vi "Version_2.0_Single_Column_Code.vi"() -> ()   [LabVIEW 2020] (continued)
                                n5689 = Subtract(x=w6119, y=w6118) -> (x-y=w6117:dbl)
                                n5690 = Absolute Value(x=w6117) -> (abs(x)=w6116:dbl)
                                n5691 = Multiply(x=w6116, y=w6115) -> (x*y=w6114:dbl)
                                n5692 = Divide(x=w6114, y=3000.0) -> (x/y=w6112:dbl)
                                }
                                frame "High Resolution Pumping".. {
                                n5693 = Subtract(x=w6127, y=w6126) -> (x-y=w6125:dbl)
                                n5694 = Absolute Value(x=w6125) -> (abs(x)=w6124:dbl)
                                n5695 = Multiply(x=w6124, y=w6123) -> (x*y=w6122:dbl)
                                n5696 = Divide(x=w6122, y=24000.0) -> (x/y=w6120:dbl)
                                }
                                }
                                n5697 = local write "True Volume being \ninjected in this\nprocess"(w6106) -> ()
                                }
                                frame #1 {
                                # "From here on 'Volume being injected \nin this process' represents the volume \nin this sub process"
                                n5698 = call "AbsolutePlungerPosition (SubVI).vi"("VISA Refnum in"=w6133) -> ("Plunger Position"=w6131:i32)  [unwired: 10 in]
                                n5699 = case shown="..\"Standard Pumping\"" w6132 {
                                tunnel: w6131 -> [w6141 w6149]
                                tunnel: w6128 -> [w6140 w6148]
                                tunnel: w6130 -> [w6137 w6145]
                                tunnel: [w6134 w6142] -> w6129
                                frame .."Standard Pumping" {
                                n5700 = Subtract(x=w6141, y=w6140) -> (x-y=w6139:dbl)
                                n5701 = Absolute Value(x=w6139) -> (abs(x)=w6138:dbl)
                                n5702 = Multiply(x=w6138, y=w6137) -> (x*y=w6136:dbl)
                                n5703 = Divide(x=w6136, y=3000.0) -> (x/y=w6134:dbl)
                                }
                                frame "High Resolution Pumping".. {
                                n5704 = Subtract(x=w6149, y=w6148) -> (x-y=w6147:dbl)
                                n5705 = Absolute Value(x=w6147) -> (abs(x)=w6146:dbl)
                                n5706 = Multiply(x=w6146, y=w6145) -> (x*y=w6144:dbl)
                                n5707 = Divide(x=w6144, y=24000.0) -> (x/y=w6142:dbl)
                                }
                                }
                                n5708 = local write "Volume being Injected \nin this process"(w6129) -> ()
                                }
                                frame #2 {
                                n5709 = local read "Discard Volume"() -> (w6153:dbl)
                                n5710 = local read "Discard fluid \nprior to 1st \ndeposition"() -> (w6158:bool)
                                n5711 = local read "Volume being Injected \nin this process"() -> (w6157:dbl)
                                n5712 = Greater Or Equal?(x=w6157, y=w6153) -> (x >= y?=w6155:bool)
                                n5713 = call "AbsolutePlungerPositionStatus (SubVI).vi"("VISA Refnum in"=w6165) -> ("read buffer"=w6164:string)  [unwired: 10 in]
                                n5714 = local read "Stop for End of \nExperiment \nand Data Writing"() -> (w6152:bool)
                                n5715 = call <vilib>:"Trim Whitespace.vi"("string"=w6164) -> ("trimmed string"=w6163:string)  [unwired: 1 in]
                                n5716 = Not(x=w6158) -> (.not. x?=w6156:bool)
                                n5717 = Equal?(x=w6163, y="/0`\u0003") -> (x = y?=w6161:bool)
                                n5718 = Or(x=w6156, y=w6155) -> (x .or. y?=w6154:bool)
                                n5719 = local read "Re-SEC"() -> (w6151:bool)
                                n5720 = Or(x=w6152, y=w6151) -> (x .or. y?=w6150:bool)
                                n5721 = Or(x=w6154, y=w6150) -> (x .or. y?=w6160:bool)
                                n5722 = Or(x=w6161, y=w6160) -> (x .or. y?=w6159:bool)
                                }
                                }
                                n5723 = Wait (ms)(milliseconds to wait=u32 100) -> ()  [unwired: 1 out]
                                }
                                n5724 = local write "Valve V4 Open"(TRUE ("Valve V4 Open")) -> ()
                                n5725 = local write "Valve V3 Open"(TRUE ("Valve V3 Open")) -> ()
                                n5726 = local write "Valve V2 Open"(FALSE ("Valve V2 Open")) -> ()
                                n5727 = local write "Valve V1 Open"(FALSE ("Valve V1 Open")) -> ()
                                n5728 = local write "External Valve \nOpen"(FALSE ("External Valve \nOpen")) -> ()
                                n5729 = local write "Valve V5 Open"(TRUE ("Valve V5 Open")) -> ()
                                n5730 = local write "Valve V6 Open"(TRUE ("Valve V6 Open")) -> ()
                                n5731 = local write "Valve V8 Open"(FALSE ("Valve V8 Open")) -> ()
                                n5732 = local write "Valve V7 Open"(FALSE ("Valve V7 Open")) -> ()
                                n5733 = local write "Volume being Injected \nin this process"(0.0) -> ()
                                }
                                frame #1 {
                                # "Keeps the on-chip valve V1, V2 and V3 closed,\nHalts also deposition onto the grid\nand waits for the 1st redeposit command. Once the command is issued\nit starts pumpoing and moves onto the next frame"
                                n5734 = stacked-sequence {
                                frame #0 {
                                n5735 = local write "Valve V5 Open"(FALSE ("Valve V5 Open")) -> ()
                                n5736 = local write "Valve V1 Open"(FALSE ("Valve V1 Open")) -> ()
                                n5737 = local read "VISA Refnum in\nfor Pump"() -> (w6177:refnum<visa-resource-name>)
                                n5738 = local write "Valve V2 Open"(FALSE ("Valve V2 Open")) -> ()
                                n5739 = local write "Valve V6 Open"(FALSE ("Valve V6 Open")) -> ()
                                n5740 = local write "Re-deposit Sample\nonto Grid"(FALSE ("Redeposit Sample\nonto Grid")) -> ()
                                n5741 = local write "Pause Data Collection"(TRUE ("Pause Data Collection")) -> ()
                                n5742 = call "HardStopCurrentProcess (SubVI).vi"("VISA Refnum in"=w6177) -> ()  [unwired: 11 in]
                                n5743 = local write "Valve V7 Open"(FALSE ("Valve V7 Open")) -> ()
                                n5744 = local write "Valve V3 Open"(FALSE ("Valve V3 Open")) -> ()
                                n5745 = local write "External Valve \nOpen"(FALSE ("External Valve \nOpen")) -> ()
                                n5746 = local write "Valve V4 Open"(FALSE ("Valve V4 Open")) -> ()
                                n5747 = local write "Valve V8 Open"(FALSE ("Valve V8 Open")) -> ()
                                }
                                frame #1 {
                                n5748 = while {
                                stop <- w6183 stop-if-true
                                n5749 = local read "Stop for End of \nExperiment \nand Data Writing"() -> (w6181:bool)
                                n5750 = local read "Re-SEC"() -> (w6182:bool)
                                n5751 = local read "Re-deposit Sample\nonto Grid"() -> (w6184:bool)
                                n5752 = Or(x=w6181, y=w6182) -> (x .or. y?=w6180:bool)
                                n5753 = Or(x=w6184, y=w6180) -> (x .or. y?=w6183:bool)
                                }
                                n5754 = local write "Discard fluid \nprior to 1st \ndeposition"(FALSE ("Discard fluid \nprior to 1st \ndeposition")) -> ()
                                n5755 = One Button Dialog(message="Do you want to deposit sample on another grid? If yes, turn on 'Re-deposit Sample onto Grid'. Else turn on Re-SEC to do SEC again or STOP to end the experiment") -> ()  [unwired: 1 in, 1 out]
                                }
                                frame #2 {
                                n5756 = local write "Valve V6 Open"(TRUE ("Valve V3 Open")) -> ()
                                n5757 = local write "Valve V4 Open"(TRUE ("Valve V1 Open")) -> ()
                                n5758 = local write "Valve V5 Open"(TRUE ("Valve V2 Open")) -> ()
                                n5759 = local write "Valve V3 Open"(TRUE ("Valve V3 Open")) -> ()
                                n5760 = local write "Valve V7 Open"(FALSE ("Valve V7 Open")) -> ()
                                }
                                frame #3 {
                                n5761 = local read "Re-deposit Sample\nonto Grid"() -> (w6190:bool)
                                n5762 = case shown="True" w6190 {
                                frame False {
                                n5763 = local write "Suction On/Off"(FALSE ("Suction On/Off")) -> ()
                                }
                                frame True {
                                n5764 = stacked-sequence {
                                frame #0 {
                                n5765 = local read "VISA Refnum in\nfor Pump"() -> (w6193:refnum<visa-resource-name>)
                                n5766 = call "AbsolutePlungerPosition (SubVI).vi"("VISA Refnum in"=w6193) -> ("Plunger Position"=w6192:i32)  [unwired: 10 in]
                                n5767 = local write "Position\nNow"(w6192) -> ()
                                }
                                frame #1 {
                                n5768 = local read "Buffer-C2 Pumping\nResolution"() -> (w6195:T2)
                                n5769 = case shown="\"Standard Pumping\", Default" w6195 {
                                tunnel: [w6196 w6207] -> w6194
                                frame "Standard Pumping", Default {
                                n5770 = local read "Buffer-C2 Volume \nto be Pumped"() -> (w6199:dbl)
                                n5771 = local read "Volume of Syringe"() -> (w6202:dbl)
                                n5772 = local read "Initial Plunger Position"() -> (w6206:dbl)
                                n5773 = local read "Position\nNow"() -> (w6205:dbl)
                                n5774 = Subtract(x=w6206, y=w6205) -> (x-y=w6204:dbl)
                                n5775 = Absolute Value(x=w6204) -> (abs(x)=w6203:dbl)
                                n5776 = Multiply(x=w6203, y=w6202) -> (x*y=w6201:dbl)
                                n5777 = Divide(x=w6201, y=3000.0) -> (x/y=w6198:dbl)
                                n5778 = Subtract(x=w6198, y=w6199) -> (x-y=w6197:dbl)
                                n5779 = Absolute Value(x=w6197) -> (abs(x)=w6196:dbl)
                                }
                                frame "High Resolution Pumping" {
                                n5780 = local read "Buffer-C2 Volume \nto be Pumped"() -> (w6210:dbl)
                                n5781 = local read "Volume of Syringe"() -> (w6213:dbl)
                                n5782 = local read "Initial Plunger Position"() -> (w6217:dbl)
                                n5783 = local read "Position\nNow"() -> (w6216:dbl)
                                n5784 = Subtract(x=w6217, y=w6216) -> (x-y=w6215:dbl)
                                n5785 = Absolute Value(x=w6215) -> (abs(x)=w6214:dbl)
                                n5786 = Multiply(x=w6214, y=w6213) -> (x*y=w6212:dbl)
                                n5787 = Divide(x=w6212, y=24000.0) -> (x/y=w6209:dbl)
                                n5788 = Subtract(x=w6209, y=w6210) -> (x-y=w6208:dbl)
                                n5789 = Absolute Value(x=w6208) -> (abs(x)=w6207:dbl)
                                }
                                }
                                n5790 = local write "Buffer-C Volume\nleft to be Pumped"(w6194) -> ()
                                }
                                frame #2 {
                                n5791 = local read "Buffer-C2 Dispense\nFlow Rate (ul/min)"() -> (w6221:dbl)
                                n5792 = local read "Buffer-C2 Pumping\nResolution"() -> (w6220:T2)
                                n5793 = local read "VISA Refnum in\nfor Pump"() -> (w6223:refnum<visa-resource-name>)
                                n5794 = local read "Volume of Syringe"() -> (w6222:dbl)
                                n5795 = call "GoToAbsolutePosition(SubVI).vi"("Absolute Volume Position in Syringe (in ul)"=0.0, "Volume of Syringe"=w6222, "Resolution of Pumping"=w6220, "Flow Rate (ul/min)"=w6221, "VISA Refnum in"=w6223) -> ()  [unwired: 6 in, 1 out]
                                n5796 = local write "Suction On/Off"(FALSE ("Suction On/Off")) -> ()
                                }
                                }
                                }
                                }
                                }
                                frame #4 {
                                n5797 = local read "Stop for End of \nExperiment \nand Data Writing"() -> (w6226:bool)
                                n5798 = local read "Re-SEC"() -> (w6225:bool)
                                n5799 = Or(x=w6226, y=w6225) -> (x .or. y?=w6224:bool)
                                n5800 = case shown="True" w6224 {
                                frame False {
                                }
                                frame True {
                                n5801 = local read "VISA Refnum in\nfor Pump"() -> (w6227:refnum<visa-resource-name>)
                                n5802 = call "HardStopCurrentProcess (SubVI).vi"("VISA Refnum in"=w6227) -> ()  [unwired: 11 in]
                                }
                                }
                                }
                                }
                                }
                                frame #2 {
                                # "Keeps the on-chip valve V1, V2 Open and V3 closed"
                                n5803 = while {
                                stop <- w6233 stop-if-true
                                n5804 = local read "Suction On/Off"() -> (w6234:bool)
                                n5805 = case shown="True" w6234 {
                                frame False {
                                n5806 = local read "Buffer-C2 Pumping\nResolution"() -> (w6240:T2)
                                n5807 = local read "Initial Plunger Position"() -> (w6239:dbl)
                                n5808 = local read "VISA Refnum in\nfor Pump"() -> (w6241:refnum<visa-resource-name>)
                                n5809 = local read "Position\nNow"() -> (w6237:dbl)
                                n5810 = local read "Volume of Syringe"() -> (w6238:dbl)
                                n5811 = local write "Volume being Injected \nin this process"(0.0) -> ()
                                n5812 = local write "Pause Data Collection"(FALSE) -> ()
                                n5813 = while {
                                tunnel: w6241 -> [w6248]
                                tunnel: w6240 -> [w6247]
                                tunnel: w6239 -> [w6243]
                                tunnel: w6238 -> [w6246]
                                tunnel: w6237 -> [w6242]
                                stop <- w6244 stop-if-true
                                n5814 = stacked-sequence {
                                tunnel: w6248 -> [w6254 w6276 w6303]
                                tunnel: w6247 -> [w6253 w6275 _]
                                tunnel: w6243 -> [w6251 _ _]
                                tunnel: w6246 -> [w6250 w6273 _]
                                tunnel: [_ _ w6296] -> w6244
                                tunnel: w6242 -> [_ w6271 _]
                                frame #0 {
                                # "From here on 'True Volume being injected \nin this process' represents the true total \nvolume in this process"
                                n5815 = call "AbsolutePlungerPosition (SubVI).vi"("VISA Refnum in"=w6254) -> ("Plunger Position"=w6252:i32)  [unwired: 10 in]
                                n5816 = case shown="..\"Standard Pumping\"" w6253 {
                                tunnel: w6252 -> [w6262 w6270]
                                tunnel: w6251 -> [w6261 w6269]
                                tunnel: w6250 -> [w6258 w6266]
                                tunnel: [w6255 w6263] -> w6249
                                frame .."Standard Pumping" {
                                n5817 = Subtract(x=w6262, y=w6261) -> (x-y=w6260:dbl)
                                n5818 = Absolute Value(x=w6260) -> (abs(x)=w6259:dbl)
                                n5819 = Multiply(x=w6259, y=w6258) -> (x*y=w6257:dbl)
                                n5820 = Divide(x=w6257, y=3000.0) -> (x/y=w6255:dbl)
                                }
                                frame "High Resolution Pumping".. {
                                n5821 = Subtract(x=w6270, y=w6269) -> (x-y=w6268:dbl)
                                n5822 = Absolute Value(x=w6268) -> (abs(x)=w6267:dbl)
                                n5823 = Multiply(x=w6267, y=w6266) -> (x*y=w6265:dbl)
                                n5824 = Divide(x=w6265, y=24000.0) -> (x/y=w6263:dbl)
                                }
                                }
                                n5825 = local write "True Volume being \ninjected in this\nprocess"(w6249) -> ()
                                }
                                frame #1 {
                                # "From here on 'Volume being injected \nin this process' represents the volume \nin this sub process"
                                n5826 = call "AbsolutePlungerPosition (SubVI).vi"("VISA Refnum in"=w6276) -> ("Plunger Position"=w6274:i32)  [unwired: 10 in]
                                n5827 = case shown="\"High Resolution Pumping\".." w6275 {
                                tunnel: w6274 -> [w6284 w6292]
                                tunnel: w6271 -> [w6283 w6291]
                                tunnel: w6273 -> [w6280 w6288]
                                tunnel: [w6277 w6285] -> w6272
                                frame .."Standard Pumping" {
                                n5828 = Subtract(x=w6284, y=w6283) -> (x-y=w6282:dbl)
                                n5829 = Absolute Value(x=w6282) -> (abs(x)=w6281:dbl)
                                n5830 = Multiply(x=w6281, y=w6280) -> (x*y=w6279:dbl)
                                n5831 = Divide(x=w6279, y=3000.0) -> (x/y=w6277:dbl)
                                }
                                frame "High Resolution Pumping".. {
                                n5832 = Subtract(x=w6292, y=w6291) -> (x-y=w6290:dbl)
                                n5833 = Absolute Value(x=w6290) -> (abs(x)=w6289:dbl)
                                n5834 = Multiply(x=w6289, y=w6288) -> (x*y=w6287:dbl)
                                n5835 = Divide(x=w6287, y=24000.0) -> (x/y=w6285:dbl)
                                }
                                }
                                n5836 = local write "Volume being Injected \nin this process"(w6272) -> ()
                                }
                                frame #2 {
                                n5837 = local read "Stop for End of \nExperiment \nand Data Writing"() -> (w6295:bool)
                                n5838 = local read "Re-SEC"() -> (w6294:bool)
                                n5839 = local read "Suction On/Off"() -> (w6299:bool)
                                n5840 = call "AbsolutePlungerPositionStatus (SubVI).vi"("VISA Refnum in"=w6303) -> ("read buffer"=w6302:string)  [unwired: 10 in]
                                n5841 = call <vilib>:"Trim Whitespace.vi"("string"=w6302) -> ("trimmed string"=w6301:string)  [unwired: 1 in]
                                n5842 = Equal?(x=w6301, y="/0`\u0003") -> (x = y?=w6298:bool)
                                n5843 = Or(x=w6295, y=w6294) -> (x .or. y?=w6293:bool)
                                n5844 = Or(x=w6299, y=w6293) -> (x .or. y?=w6297:bool)
                                n5845 = Or(x=w6298, y=w6297) -> (x .or. y?=w6296:bool)
                                }
                                }
                                n5846 = Wait (ms)(milliseconds to wait=u32 100) -> ()  [unwired: 1 out]
                                }
                                }
                                frame True {
                                n5847 = stacked-sequence {
                                frame #0 {
                                n5848 = local write "Valve V3 Open"(FALSE ("Valve V3 Open")) -> ()
                                n5849 = local read "Suction Pressure\nfor EM-grid \nDeposition (mbar)"() -> (w6310:sgl)
                                n5850 = local write "Valve V4 Open"(FALSE ("Valve V4 Open")) -> ()
                                n5851 = local read "VISA Refnum in\nfor Pump"() -> (w6313:refnum<visa-resource-name>)
                                n5852 = local write "Valve V5 Open"(FALSE ("Valve V1 Open")) -> ()
                                n5853 = local write "Suction pressure \nfor grid deposition"(w6310) -> ()
                                n5854 = local write "Re-deposit Sample\nonto Grid"(FALSE ("Redeposit Sample\nonto Grid")) -> ()
                                n5855 = local write "Pause Data Collection"(TRUE ("Pause Data Collection")) -> ()
                                n5856 = call "HardStopCurrentProcess (SubVI).vi"("VISA Refnum in"=w6313) -> ()  [unwired: 11 in]
                                n5857 = local write "Valve V6 Open"(TRUE ("Valve V2 Open")) -> ()
                                n5858 = local write "Valve V7 Open"(TRUE ("Valve V3 Open")) -> ()
                                n5859 = local write "External Valve \nOpen"(FALSE ("External Valve \nOpen")) -> ()
                                }
                                frame #1 {
                                n5860 = while {
                                stop <- w6316 stop-if-true
                                n5861 = local read "Stop for End of \nExperiment \nand Data Writing"() -> (w6317:bool)
                                n5862 = local read "Suction Pressure\nfor EM-grid \nDeposition (mbar)"() -> (w6314:sgl)
                                n5863 = call <vilib>:"fgt set pressure.vi"("pressure"=w6314, "pressureIndex"=u32 1) -> ()  [unwired: 9 in, 1 out]
                                n5864 = local read "Suction On/Off"() -> (w6319:bool)
                                n5865 = Not(x=w6319) -> (.not. x?=w6318:bool)
                                n5866 = Wait (ms)(milliseconds to wait=u32 100) -> ()  [unwired: 1 out]
                                n5867 = Or(x=w6318, y=w6317) -> (x .or. y?=w6316:bool)
                                }
                                }
                                frame #2 {
                                n5868 = for {
                                N: 2 -> [_]
                                n5869 = while {
                                stop <- w6329 stop-if-true
                                n5870 = local read "Stop for End of \nExperiment \nand Data Writing"() -> (w6325:bool)
                                n5871 = local read "Suction On/Off"() -> (w6327:bool)
                                n5872 = call <vilib>:"fgt set pressure.vi"("pressure"=sgl 0.0, "pressureIndex"=u32 1) -> ()  [unwired: 9 in, 1 out]
                                n5873 = Not(x=w6327) -> (.not. x?=w6326:bool)
                                n5874 = Wait (ms)(milliseconds to wait=u32 100) -> ()  [unwired: 1 out]
                                n5875 = Or(x=w6326, y=w6325) -> (x .or. y?=w6329:bool)
                                }
                                n5876 = Wait (ms)(milliseconds to wait=u32 400) -> ()  [unwired: 1 out]
                                }
                                }
                                frame #3 {
                                n5877 = local read "Automatic purging \nof capillary after \ngrid deposition"() -> (w6330:bool)
                                n5878 = case shown="True" w6330 {
                                frame False {
                                }
                                frame True {
                                n5879 = stacked-sequence {
                                frame #0 {
                                n5880 = local read "VISA Refnum in\nfor Pump"() -> (w6332:refnum<visa-resource-name>)
                                n5881 = call "AbsolutePlungerPosition (SubVI).vi"("VISA Refnum in"=w6332) -> ("Plunger Position"=w6331:i32)  [unwired: 10 in]
                                n5882 = local write "Position\nNow"(w6331) -> ()
                                }
                                frame #1 {
                                n5883 = local read "Buffer-C2 Pumping\nResolution"() -> (w6334:T2)
                                n5884 = case shown="\"Standard Pumping\", Default" w6334 {
                                tunnel: [w6335 w6346] -> w6333
                                frame "Standard Pumping", Default {
                                n5885 = local read "Buffer-C2 Volume \nto be Pumped"() -> (w6338:dbl)
                                n5886 = local read "Volume of Syringe"() -> (w6341:dbl)
                                n5887 = local read "Initial Plunger Position"() -> (w6345:dbl)
                                n5888 = local read "Position\nNow"() -> (w6344:dbl)
                                n5889 = Subtract(x=w6345, y=w6344) -> (x-y=w6343:dbl)
                                n5890 = Absolute Value(x=w6343) -> (abs(x)=w6342:dbl)
                                n5891 = Multiply(x=w6342, y=w6341) -> (x*y=w6340:dbl)
                                n5892 = Divide(x=w6340, y=3000.0) -> (x/y=w6337:dbl)
                                n5893 = Subtract(x=w6337, y=w6338) -> (x-y=w6336:dbl)
                                n5894 = Absolute Value(x=w6336) -> (abs(x)=w6335:dbl)
                                }
                                frame "High Resolution Pumping" {
                                n5895 = local read "Buffer-C2 Volume \nto be Pumped"() -> (w6349:dbl)
                                n5896 = local read "Volume of Syringe"() -> (w6352:dbl)
                                n5897 = local read "Initial Plunger Position"() -> (w6356:dbl)
                                n5898 = local read "Position\nNow"() -> (w6355:dbl)
                                n5899 = Subtract(x=w6356, y=w6355) -> (x-y=w6354:dbl)
                                n5900 = Absolute Value(x=w6354) -> (abs(x)=w6353:dbl)
                                n5901 = Multiply(x=w6353, y=w6352) -> (x*y=w6351:dbl)
                                n5902 = Divide(x=w6351, y=24000.0) -> (x/y=w6348:dbl)
                                n5903 = Subtract(x=w6348, y=w6349) -> (x-y=w6347:dbl)
                                n5904 = Absolute Value(x=w6347) -> (abs(x)=w6346:dbl)
                                }
                                }
                                n5905 = local write "Buffer-C Volume\nleft to be Pumped"(w6333) -> ()
                                }
                                frame #2 {
                                n5906 = local read "Buffer-C2 Dispense\nFlow Rate (ul/min)"() -> (w6365:dbl)
                                n5907 = local read "Buffer-C2 Pumping\nResolution"() -> (w6364:T2)
                                n5908 = local read "VISA Refnum in\nfor Pump"() -> (w6367:refnum<visa-resource-name>)
                                n5909 = local read "Volume of Syringe"() -> (w6366:dbl)
                                n5910 = call "GoToAbsolutePosition(SubVI).vi"("Absolute Volume Position in Syringe (in ul)"=0.0, "Volume of Syringe"=w6366, "Resolution of Pumping"=w6364, "Flow Rate (ul/min)"=w6365, "VISA Refnum in"=w6367) -> ()  [unwired: 6 in, 1 out]
                                n5911 = local write "External Valve \nOpen"(FALSE ("External Valve \nOpen")) -> ()
                                n5912 = local write "Valve V3 Open"(TRUE ("Valve V3 Open")) -> ()
                                n5913 = local write "Valve V7 Open"(FALSE ("Valve V3 Open")) -> ()
                                n5914 = local write "Valve V5 Open"(TRUE ("Valve V1 Open")) -> ()
                                n5915 = local write "Valve V6 Open"(TRUE ("Valve V2 Open")) -> ()
                                n5916 = local write "Valve V4 Open"(TRUE ("Valve V4 Open")) -> ()
                                }
                                frame #3 {
                                n5917 = local read "Buffer-C2 Pumping\nResolution"() -> (w6373:T2)
                                n5918 = local read "Initial Plunger Position"() -> (w6372:dbl)
                                n5919 = local read "VISA Refnum in\nfor Pump"() -> (w6374:refnum<visa-resource-name>)
                                n5920 = local read "Position\nNow"() -> (w6370:dbl)
                                n5921 = local read "Volume of Syringe"() -> (w6371:dbl)
                                n5922 = local write "Volume being Injected \nin this process"(0.0) -> ()
                                n5923 = local write "Pause Data Collection"(FALSE) -> ()
                                n5924 = while {
                                tunnel: w6374 -> [w6381]
                                tunnel: w6373 -> [w6380]
                                tunnel: w6372 -> [w6376]
                                tunnel: w6371 -> [w6379]
                                tunnel: w6370 -> [w6375]
                                stop <- w6377 stop-if-true
                                n5925 = stacked-sequence {
                                tunnel: w6381 -> [w6387 w6409 w6438]
                                tunnel: w6380 -> [w6386 w6408 _]
                                tunnel: w6376 -> [w6384 _ _]
                                tunnel: w6379 -> [w6383 w6406 _]
                                tunnel: [_ _ w6432] -> w6377
                                tunnel: w6375 -> [_ w6404 _]
                                frame #0 {
                                # "From here on 'True Volume being injected \nin this process' represents the true total \nvolume in this process"
                                n5926 = call "AbsolutePlungerPosition (SubVI).vi"("VISA Refnum in"=w6387) -> ("Plunger Position"=w6385:i32)  [unwired: 10 in]
                                n5927 = case shown="..\"Standard Pumping\"" w6386 {
                                tunnel: w6385 -> [w6395 w6403]
                                tunnel: w6384 -> [w6394 w6402]
                                tunnel: w6383 -> [w6391 w6399]
                                tunnel: [w6388 w6396] -> w6382
                                frame .."Standard Pumping" {
                                n5928 = Subtract(x=w6395, y=w6394) -> (x-y=w6393:dbl)
                                n5929 = Absolute Value(x=w6393) -> (abs(x)=w6392:dbl)
                                n5930 = Multiply(x=w6392, y=w6391) -> (x*y=w6390:dbl)
                                n5931 = Divide(x=w6390, y=3000.0) -> (x/y=w6388:dbl)
                                }
                                frame "High Resolution Pumping".. {
                                n5932 = Subtract(x=w6403, y=w6402) -> (x-y=w6401:dbl)
                                n5933 = Absolute Value(x=w6401) -> (abs(x)=w6400:dbl)
                                n5934 = Multiply(x=w6400, y=w6399) -> (x*y=w6398:dbl)
                                n5935 = Divide(x=w6398, y=24000.0) -> (x/y=w6396:dbl)
                                }
                                }
                                n5936 = local write "True Volume being \ninjected in this\nprocess"(w6382) -> ()
                                }
                                frame #1 {
                                # "From here on 'Volume being injected \nin this process' represents the volume \nin this sub process"
                                n5937 = call "AbsolutePlungerPosition (SubVI).vi"("VISA Refnum in"=w6409) -> ("Plunger Position"=w6407:i32)  [unwired: 10 in]
                                n5938 = case shown="\"High Resolution Pumping\".." w6408 {
                                tunnel: w6407 -> [w6417 w6425]
                                tunnel: w6404 -> [w6416 w6424]
                                tunnel: w6406 -> [w6413 w6421]
                                tunnel: [w6410 w6418] -> w6405
                                frame .."Standard Pumping" {
                                n5939 = Subtract(x=w6417, y=w6416) -> (x-y=w6415:dbl)
                                n5940 = Absolute Value(x=w6415) -> (abs(x)=w6414:dbl)
                                n5941 = Multiply(x=w6414, y=w6413) -> (x*y=w6412:dbl)
                                n5942 = Divide(x=w6412, y=3000.0) -> (x/y=w6410:dbl)
                                }
                                frame "High Resolution Pumping".. {
                                n5943 = Subtract(x=w6425, y=w6424) -> (x-y=w6423:dbl)
                                n5944 = Absolute Value(x=w6423) -> (abs(x)=w6422:dbl)
                                n5945 = Multiply(x=w6422, y=w6421) -> (x*y=w6420:dbl)
                                n5946 = Divide(x=w6420, y=24000.0) -> (x/y=w6418:dbl)
                                }
                                }
                                n5947 = local write "Volume being Injected \nin this process"(w6405) -> ()
                                }
                                frame #2 {
                                n5948 = local read "Capillary purge \nvolume after every\ngrid plunging"() -> (w6427:dbl)
                                n5949 = local read "Stop for End of \nExperiment \nand Data Writing"() -> (w6431:bool)
                                n5950 = local read "Volume being Injected \nin this process"() -> (w6428:dbl)
                                n5951 = local read "Re-SEC"() -> (w6430:bool)
                                n5952 = call "AbsolutePlungerPositionStatus (SubVI).vi"("VISA Refnum in"=w6438) -> ("read buffer"=w6437:string)  [unwired: 10 in]
                                n5953 = call <vilib>:"Trim Whitespace.vi"("string"=w6437) -> ("trimmed string"=w6436:string)  [unwired: 1 in]
                                n5954 = Greater Or Equal?(x=w6428, y=w6427) -> (x >= y?=w6426:bool)
                                n5955 = Equal?(x=w6436, y="/0`\u0003") -> (x = y?=w6434:bool)
                                n5956 = Or(x=w6431, y=w6430) -> (x .or. y?=w6429:bool)
                                n5957 = Or(x=w6426, y=w6429) -> (x .or. y?=w6433:bool)
                                n5958 = Or(x=w6434, y=w6433) -> (x .or. y?=w6432:bool)
                                }
                                }
                                n5959 = Wait (ms)(milliseconds to wait=u32 100) -> ()  [unwired: 1 out]
                                }
                                }
                                frame #4 {
                                n5960 = local read "VISA Refnum in\nfor Pump"() -> (w6439:refnum<visa-resource-name>)
                                n5961 = call "HardStopCurrentProcess (SubVI).vi"("VISA Refnum in"=w6439) -> ()  [unwired: 11 in]
                                }
                                }
                                }
                                }
                                }
                                frame #4 {
                                n5962 = local write "Valve V3 Open"(FALSE ("Valve V3 Open")) -> ()
                                n5963 = local write "Valve V7 Open"(FALSE ("Valve V3 Open")) -> ()
                                n5964 = local write "Valve V5 Open"(FALSE ("Valve V1 Open")) -> ()
                                n5965 = local write "Valve V6 Open"(FALSE ("Valve V2 Open")) -> ()
                                n5966 = local write "Valve V4 Open"(FALSE ("Valve V4 Open")) -> ()
                                }
                                frame #5 {
                                n5967 = while {
                                stop <- w6449 stop-if-true
                                n5968 = local read "Stop for End of \nExperiment \nand Data Writing"() -> (w6447:bool)
                                n5969 = local read "Re-deposit Sample\nonto Grid"() -> (w6450:bool)
                                n5970 = local read "Re-SEC"() -> (w6448:bool)
                                n5971 = Or(x=w6447, y=w6448) -> (x .or. y?=w6446:bool)
                                n5972 = Or(x=w6450, y=w6446) -> (x .or. y?=w6449:bool)
                                }
                                n5973 = One Button Dialog(message="Do you want to deposit sample on another grid? If yes, turn on 'Re-deposit Sample onto Grid'. Else turn on Re-SEC to do SEC again or STOP to end the experiment") -> ()  [unwired: 1 in, 1 out]
                                }
                                frame #6 {
                                n5974 = local write "Valve V4 Open"(TRUE ("Valve V4 Open")) -> ()
                                n5975 = local write "Valve V3 Open"(TRUE ("Valve V3 Open")) -> ()
                                n5976 = local write "Valve V7 Open"(FALSE ("Valve V3 Open")) -> ()
                                n5977 = local write "Valve V5 Open"(TRUE ("Valve V1 Open")) -> ()
                                n5978 = local write "Valve V6 Open"(TRUE ("Valve V2 Open")) -> ()
                                }
                                frame #7 {
                                n5979 = local read "Re-deposit Sample\nonto Grid"() -> (w6456:bool)
                                n5980 = case shown="True" w6456 {
                                frame False {
                                n5981 = local write "Suction On/Off"(FALSE ("Suction On/Off")) -> ()
                                }
                                frame True {
                                n5982 = stacked-sequence {
                                frame #0 {
                                n5983 = local read "VISA Refnum in\nfor Pump"() -> (w6459:refnum<visa-resource-name>)
                                n5984 = call "AbsolutePlungerPosition (SubVI).vi"("VISA Refnum in"=w6459) -> ("Plunger Position"=w6458:i32)  [unwired: 10 in]
                                n5985 = local write "Position\nNow"(w6458) -> ()
                                }
                                frame #1 {
                                n5986 = local read "Buffer-C2 Pumping\nResolution"() -> (w6461:T2)
                                n5987 = case shown="\"Standard Pumping\", Default" w6461 {
                                tunnel: [w6462 w6473] -> w6460
                                frame "Standard Pumping", Default {
                                n5988 = local read "Buffer-C2 Volume \nto be Pumped"() -> (w6465:dbl)
                                n5989 = local read "Volume of Syringe"() -> (w6468:dbl)
                                n5990 = local read "Initial Plunger Position"() -> (w6472:dbl)
                                n5991 = local read "Position\nNow"() -> (w6471:dbl)
                                n5992 = Subtract(x=w6472, y=w6471) -> (x-y=w6470:dbl)
                                n5993 = Absolute Value(x=w6470) -> (abs(x)=w6469:dbl)
                                n5994 = Multiply(x=w6469, y=w6468) -> (x*y=w6467:dbl)
                                n5995 = Divide(x=w6467, y=3000.0) -> (x/y=w6464:dbl)
                                n5996 = Subtract(x=w6464, y=w6465) -> (x-y=w6463:dbl)
                                n5997 = Absolute Value(x=w6463) -> (abs(x)=w6462:dbl)
                                }
                                frame "High Resolution Pumping" {
                                n5998 = local read "Buffer-C2 Volume \nto be Pumped"() -> (w6476:dbl)
                                n5999 = local read "Volume of Syringe"() -> (w6479:dbl)
                                n6000 = local read "Initial Plunger Position"() -> (w6483:dbl)
                                n6001 = local read "Position\nNow"() -> (w6482:dbl)
                                n6002 = Subtract(x=w6483, y=w6482) -> (x-y=w6481:dbl)
                                n6003 = Absolute Value(x=w6481) -> (abs(x)=w6480:dbl)
                                n6004 = Multiply(x=w6480, y=w6479) -> (x*y=w6478:dbl)
                                n6005 = Divide(x=w6478, y=24000.0) -> (x/y=w6475:dbl)
                                n6006 = Subtract(x=w6475, y=w6476) -> (x-y=w6474:dbl)
                                n6007 = Absolute Value(x=w6474) -> (abs(x)=w6473:dbl)
                                }
                                }
                                n6008 = local write "Buffer-C Volume\nleft to be Pumped"(w6460) -> ()
                                }
                                frame #2 {
                                n6009 = local read "Buffer-C2 Dispense\nFlow Rate (ul/min)"() -> (w6487:dbl)
                                n6010 = local read "Buffer-C2 Pumping\nResolution"() -> (w6486:T2)
                                n6011 = local read "VISA Refnum in\nfor Pump"() -> (w6489:refnum<visa-resource-name>)
                                n6012 = local read "Volume of Syringe"() -> (w6488:dbl)
                                n6013 = call "GoToAbsolutePosition(SubVI).vi"("Absolute Volume Position in Syringe (in ul)"=0.0, "Volume of Syringe"=w6488, "Resolution of Pumping"=w6486, "Flow Rate (ul/min)"=w6487, "VISA Refnum in"=w6489) -> ()  [unwired: 6 in, 1 out]
                                n6014 = local write "Suction On/Off"(FALSE ("Suction On/Off")) -> ()
                                }
                                }
                                }
                                }
                                }
                                frame #8 {
                                n6015 = local read "Stop for End of \nExperiment \nand Data Writing"() -> (w6491:bool)
                                n6016 = local read "Re-SEC"() -> (w6492:bool)
                                n6017 = Or(x=w6491, y=w6492) -> (x .or. y?=w6490:bool)
                                n6018 = case shown="True" w6490 {
                                frame False {
                                }
                                frame True {
                                n6019 = local read "VISA Refnum in\nfor Pump"() -> (w6493:refnum<visa-resource-name>)
                                n6020 = call "HardStopCurrentProcess (SubVI).vi"("VISA Refnum in"=w6493) -> ()  [unwired: 11 in]
                                }
                                }
                                }
                                }
                                }
                                }
                                n6021 = local read "Stop for End of \nExperiment \nand Data Writing"() -> (w6229:bool)
                                n6022 = local read "Divert Sample \nonto Grid"() -> (w6232:bool)
                                n6023 = local read "Re-SEC"() -> (w6230:bool)
                                n6024 = Not(x=w6232) -> (.not. x?=w6231:bool)
                                n6025 = Or(x=w6229, y=w6230) -> (x .or. y?=w6228:bool)
                                n6026 = Or(x=w6231, y=w6228) -> (x .or. y?=w6233:bool)
                                }
                                }
                                }
                                n6027 = local write "Discard fluid \nprior to 1st \ndeposition"(TRUE ("Discard fluid \nprior to 1st \ndeposition")) -> ()
                              }
                            }
                          }
                          frame #34 {
                            n6028 = local read "Stopper that ends \nthe main loops"() -> (w6495:bool)
                            n6029 = local read "Re-SEC"() -> (w6496:bool)
                            n6030 = Wait (ms)(milliseconds to wait=u32 500) -> ()  [unwired: 1 out]
                            n6031 = Or(x=w6495, y=w6496) -> (x .or. y?=w6494:bool)
                            n6032 = case shown="True" w6494 {
                              frame False {
                              }
                              frame True {
                                n6033 = local read "VISA Refnum in\nfor Pump"() -> (w6501:refnum<visa-resource-name>)
                                n6034 = call "HardStopCurrentProcess (SubVI).vi"("VISA Refnum in"=w6501) -> ()  [unwired: 11 in]
                              }
                            }
                            n6035 = local write "Divert Sample \nonto Grid"(FALSE ("Divert Sample \nonto Grid")) -> ()
                            n6036 = local write "Pause Data Collection"(TRUE ("Pause Data Collection")) -> ()
                            n6037 = local write "Start the Process"(FALSE ("Start the Process")) -> ()
                          }
                          frame #35 {
                            n6038 = local read "Stop for End of \nExperiment \nand Data Writing"() -> (w6508:bool)
                            n6039 = local read "Start the Process"() -> (w6507:bool)
                            n6040 = Or(x=w6507, y=w6508) -> (x .or. y?=w6506:bool)
                            n6041 = case shown="False" w6506 {
                              frame False {
                                n6042 = while {
                                stop <- w6514 stop-if-true
                                n6043 = local read "Stop for End of \nExperiment \nand Data Writing"() -> (w6516:bool)
                                n6044 = local read "Start the Process"() -> (w6515:bool)
                                n6045 = Or(x=w6515, y=w6516) -> (x .or. y?=w6514:bool)
                                n6046 = Wait (ms)(milliseconds to wait=u32 100) -> ()  [unwired: 1 out]
                                }
                                n6047 = One Button Dialog(message="Do you want to re-introduce sample into column-2 and elute? If yes, adjust the re-introduction volume into column-2 and elution parameters for column-2 and turn on the 'Start the Process' button . If no, turn on the 'Stop for End of Experiment and Data Writing'.") -> ()  [unwired: 1 in, 1 out]
                              }
                              frame True {
                                n6048 = local read "Stop for End of \nExperiment \nand Data Writing"() -> (w6517:bool)
                                n6049 = case shown="True" w6517 {
                                frame False {
                                }
                                frame True {
                                n6050 = local write "Valve V1 Open"(FALSE ("Valve V1 Open")) -> ()
                                n6051 = local write "Valve V2 Open"(FALSE ("Valve V2 Open")) -> ()
                                n6052 = local write "Valve V4 Open"(FALSE ("Valve V4 Open")) -> ()
                                n6053 = local write "Valve V3 Open"(FALSE ("Valve V3 Open")) -> ()
                                n6054 = local write "Valve V5 Open"(FALSE ("Valve V5 Open")) -> ()
                                n6055 = local write "Valve V6 Open"(FALSE ("Valve V6 Open")) -> ()
                                n6056 = local write "Valve V7 Open"(FALSE ("Valve V7 Open")) -> ()
                                }
                                }
                              }
                            }
                            n6057 = local write "Sample Volume Diverted\ninto Column-2"(0.0 ("Sample Volume Diverted\ninto Column-2")) -> ()
                            n6058 = local write "Buffer-C Volume\nleft to be Pumped"(0.0 ("Buffer-C Volume\nleft to be Pumped")) -> ()
                            n6059 = local write "Vol_previous"(0.0 ("Vol_previous")) -> ()
                            n6060 = local write "Vol_now"(0.0 ("Vol_now")) -> ()
                            n6061 = local write "Elution of Column-2"(FALSE ("Elution of Column-2")) -> ()
                            n6062 = local write "SEC On"(FALSE ("SEC On")) -> ()
                            n6063 = local write "Volume being Injected \nin this process"(0.0 ("Volume being Injected \nin this process")) -> ()
                          }
                        }
                      }
                      frame #5 {
                        n6064 = while {
                          stop <- w6526 stop-if-true
                          # "Re-introduce Sample into Column-2, Elute column-2 and Divert the sample onto Grid"
                          n6065 = local read "Start the Process"() -> (w6525:bool)
                          n6066 = case shown="True" w6525 {
                            frame False {
                            }
                            frame True {
                              n6067 = stacked-sequence {
                                frame #0 {
                                # "Reinitialize the pump"
                                n6068 = local read "VISA Refnum in\nfor Pump"() -> (w6528:refnum<visa-resource-name>)
                                n6069 = call "Initializer (SubVI).vi"("VISA Refnum in"=w6528) -> ()  [unwired: 11 in]
                                n6070 = local write "Re-SEC"(FALSE ("Re-SEC")) -> ()
                                }
                                frame #1 {
                                # "If Yes, this code will clean the column-2 with buffer-C prior to re-introducing the sample"
                                n6071 = local read "Wash column-2 Prior \nto re-introducing \nsample"() -> (w6529:bool)
                                n6072 = case shown="True" w6529 {
                                frame False {
                                }
                                frame True {
                                n6073 = stacked-sequence {
                                frame #0 {
                                n6074 = local read "VISA Refnum in\nfor Pump"() -> (w6531:refnum<visa-resource-name>)
                                n6075 = local read "Port for \nC2-Elution"() -> (w6530:string)
                                n6076 = call "PortChanger (SubVI).vi"("Port Number"=w6530, "VISA Refnum in"=w6531) -> ()  [unwired: 10 in]
                                }
                                frame #1 {
                                n6077 = local read "Stopper that ends \nthe main loops"() -> (w6532:bool)
                                n6078 = local read "VISA Refnum in\nfor Pump"() -> (w6533:refnum<visa-resource-name>)
                                n6079 = case shown="True" w6532 {
                                frame False {
                                }
                                frame True {
                                n6080 = local read "VISA Refnum in\nfor Pump"() -> (w6534:refnum<visa-resource-name>)
                                n6081 = call "HardStopCurrentProcess (SubVI).vi"("VISA Refnum in"=w6534) -> ()  [unwired: 11 in]
                                }
                                }
                                n6082 = call "ProcessCompletionWaiter (SubVI).vi"("VISA Refnum in"=w6533) -> ()  [unwired: 11 in]
                                }
                                frame #2 {
                                n6083 = local read "Buffer-B Pumping\nResolution"() -> (w6537:T2)
                                n6084 = local read "VISA Refnum in\nfor Pump"() -> (w6539:refnum<visa-resource-name>)
                                n6085 = local read "Buffer-C2 \nWash Volume\nPrior to re-introducing \nSample"() -> (w6536:dbl)
                                n6086 = local read "Volume of Syringe"() -> (w6538:dbl)
                                n6087 = call "RPickUp(SubVI).vi"("Volume to be picked up"=w6536, "Volume of Syringe"=w6538, "Resolution of PickUP"=w6537, "PickUp Flow Rate (ul/min)"=150.0, "VISA Refnum in"=w6539) -> ()  [unwired: 6 in, 1 out]
                                }
                                frame #3 {
                                n6088 = local read "Stopper that ends \nthe main loops"() -> (w6540:bool)
                                n6089 = local read "VISA Refnum in\nfor Pump"() -> (w6541:refnum<visa-resource-name>)
                                n6090 = case shown="True" w6540 {
                                frame False {
                                }
                                frame True {
                                n6091 = local read "VISA Refnum in\nfor Pump"() -> (w6542:refnum<visa-resource-name>)
                                n6092 = call "HardStopCurrentProcess (SubVI).vi"("VISA Refnum in"=w6542) -> ()  [unwired: 11 in]
                                }
                                }
                                n6093 = call "ProcessCompletionWaiter (SubVI).vi"("VISA Refnum in"=w6541) -> ()  [unwired: 11 in]
                                }
                                frame #4 {
                                n6094 = local read "VISA Refnum in\nfor Pump"() -> (w6544:refnum<visa-resource-name>)
                                n6095 = call "PortChanger (SubVI).vi"("Port Number"="10", "VISA Refnum in"=w6544) -> ()  [unwired: 10 in]
                                }
                                frame #5 {
                                n6096 = local read "Stopper that ends \nthe main loops"() -> (w6545:bool)
                                n6097 = local read "VISA Refnum in\nfor Pump"() -> (w6546:refnum<visa-resource-name>)
                                n6098 = case shown="True" w6545 {
                                frame False {
                                }
                                frame True {
                                n6099 = local read "VISA Refnum in\nfor Pump"() -> (w6547:refnum<visa-resource-name>)
                                n6100 = call "HardStopCurrentProcess (SubVI).vi"("VISA Refnum in"=w6547) -> ()  [unwired: 11 in]
                                }
                                }
                                n6101 = call "ProcessCompletionWaiter (SubVI).vi"("VISA Refnum in"=w6546) -> ()  [unwired: 11 in]
                                }
                                frame #6 {
                                n6102 = local read "Buffer-C2 Dispense \nFlow Rate for Washing \nPrior to re-introducing Sample"() -> (w6548:dbl)
                                n6103 = local read "VISA Refnum in\nfor Pump"() -> (w6552:refnum<visa-resource-name>)
                                n6104 = local read "Volume of Syringe"() -> (w6550:dbl)
                                n6105 = call "GoToAbsolutePosition(SubVI).vi"("Absolute Volume Position in Syringe (in ul)"=0.0, "Volume of Syringe"=w6550, "Resolution of Pumping"=T2."Standard Pumping", "Flow Rate (ul/min)"=w6548, "VISA Refnum in"=w6552) -> ()  [unwired: 6 in, 1 out]
                                }
                                frame #7 {
                                n6106 = local read "Stopper that ends \nthe main loops"() -> (w6553:bool)
                                n6107 = local read "VISA Refnum in\nfor Pump"() -> (w6554:refnum<visa-resource-name>)
                                n6108 = case shown="True" w6553 {
                                frame False {
                                }
                                frame True {
                                n6109 = local read "VISA Refnum in\nfor Pump"() -> (w6555:refnum<visa-resource-name>)
                                n6110 = call "HardStopCurrentProcess (SubVI).vi"("VISA Refnum in"=w6555) -> ()  [unwired: 11 in]
                                }
                                }
                                n6111 = call "ProcessCompletionWaiter (SubVI).vi"("VISA Refnum in"=w6554) -> ()  [unwired: 11 in]
                                }
                                }
                                }
                                }
                                }
                                frame #2 {
                                # "Switch to Port-7"
                                # "Port-7 of pump is connected to Buffer-B"
                                n6112 = local write "Washing Column-2"(FALSE ("Washing Column-2")) -> ()
                                n6113 = local read "VISA Refnum in\nfor Pump"() -> (w6562:refnum<visa-resource-name>)
                                n6114 = local read "Port for \nB-Elution"() -> (w6560:string)
                                n6115 = local write "Affinity Elution On"(TRUE ("Affinity Elution On")) -> ()
                                n6116 = call "PortChanger (SubVI).vi"("Port Number"=w6560, "VISA Refnum in"=w6562) -> ()  [unwired: 10 in]
                                n6117 = local write "Elution of Column-1"(TRUE ("Elution of Column-1")) -> ()
                                n6118 = local write "Clean the \nBuffer-B tubing"(FALSE ("Clean the \nBuffer-B tubing")) -> ()
                                n6119 = local write "Divert Sample \ninto Column-2"(TRUE ("Divert Sample \ninto Column-2")) -> ()
                                }
                                frame #3 {
                                n6120 = local read "VISA Refnum in\nfor Pump"() -> (w6563:refnum<visa-resource-name>)
                                n6121 = call "ProcessCompletionWaiter (SubVI).vi"("VISA Refnum in"=w6563) -> ()  [unwired: 11 in]
                                }
                                frame #4 {
                                # "If Yes, it will clean the elution buffer from port-5 tubing a bit more"
                                n6122 = local read "Clean the \nBuffer-B tubing"() -> (w6564:bool)
                                n6123 = case shown="True" w6564 {
                                frame False {
                                n6124 = stacked-sequence {
                                frame #0 {
                                n6125 = local read "Buffer-B Pumping\nResolution"() -> (w6567:T2)
                                n6126 = local read "VISA Refnum in\nfor Pump"() -> (w6569:refnum<visa-resource-name>)
                                n6127 = local read "V-S"() -> (w6566:dbl)
                                n6128 = local read "Volume of Syringe"() -> (w6568:dbl)
                                n6129 = call "RPickUp(SubVI).vi"("Volume to be picked up"=w6566, "Volume of Syringe"=w6568, "Resolution of PickUP"=w6567, "PickUp Flow Rate (ul/min)"=150.0, "VISA Refnum in"=w6569) -> ()  [unwired: 6 in, 1 out]
                                }
                                frame #1 {
                                n6130 = local read "Stopper that ends \nthe main loops"() -> (w6570:bool)
                                n6131 = local read "VISA Refnum in\nfor Pump"() -> (w6571:refnum<visa-resource-name>)
                                n6132 = case shown="True" w6570 {
                                frame False {
                                }
                                frame True {
                                n6133 = local read "VISA Refnum in\nfor Pump"() -> (w6572:refnum<visa-resource-name>)
                                n6134 = call "HardStopCurrentProcess (SubVI).vi"("VISA Refnum in"=w6572) -> ()  [unwired: 11 in]
                                }
                                }
                                n6135 = call "ProcessCompletionWaiter (SubVI).vi"("VISA Refnum in"=w6571) -> ()  [unwired: 11 in]
                                }
                                frame #2 {
                                n6136 = local read "VISA Refnum in\nfor Pump"() -> (w6574:refnum<visa-resource-name>)
                                n6137 = call "PortChanger (SubVI).vi"("Port Number"="1", "VISA Refnum in"=w6574) -> ()  [unwired: 10 in]
                                }
                                frame #3 {
                                n6138 = local read "Stopper that ends \nthe main loops"() -> (w6575:bool)
                                n6139 = local read "VISA Refnum in\nfor Pump"() -> (w6576:refnum<visa-resource-name>)
                                n6140 = case shown="True" w6575 {
                                frame False {
                                }
                                frame True {
                                n6141 = local read "VISA Refnum in\nfor Pump"() -> (w6577:refnum<visa-resource-name>)
                                n6142 = call "HardStopCurrentProcess (SubVI).vi"("VISA Refnum in"=w6577) -> ()  [unwired: 11 in]
                                }
                                }
                                n6143 = call "ProcessCompletionWaiter (SubVI).vi"("VISA Refnum in"=w6576) -> ()  [unwired: 11 in]
                                }
                                frame #4 {
                                n6144 = local read "VISA Refnum in\nfor Pump"() -> (w6582:refnum<visa-resource-name>)
                                n6145 = local read "Volume of Syringe"() -> (w6579:dbl)
                                n6146 = call "GoToAbsolutePosition(SubVI).vi"("Absolute Volume Position in Syringe (in ul)"=0.0, "Volume of Syringe"=w6579, "Resolution of Pumping"=T2."Standard Pumping", "Flow Rate (ul/min)"=150.0, "VISA Refnum in"=w6582) -> ()  [unwired: 6 in, 1 out]
                                }
                                frame #5 {
                                n6147 = local read "Stopper that ends \nthe main loops"() -> (w6583:bool)
                                n6148 = local read "VISA Refnum in\nfor Pump"() -> (w6584:refnum<visa-resource-name>)
                                n6149 = case shown="True" w6583 {
                                frame False {
                                }
                                frame True {
                                n6150 = local read "VISA Refnum in\nfor Pump"() -> (w6585:refnum<visa-resource-name>)
                                n6151 = call "HardStopCurrentProcess (SubVI).vi"("VISA Refnum in"=w6585) -> ()  [unwired: 11 in]
                                }
                                }
                                n6152 = call "ProcessCompletionWaiter (SubVI).vi"("VISA Refnum in"=w6584) -> ()  [unwired: 11 in]
                                }
                                }
                                }
                                frame True {
                                n6153 = for {
                                N: 2 -> [_]
                                n6154 = stacked-sequence {
                                frame #0 {
                                n6155 = local read "Buffer-B Pumping\nResolution"() -> (w6589:T2)
                                n6156 = local read "VISA Refnum in\nfor Pump"() -> (w6591:refnum<visa-resource-name>)
                                n6157 = local read "Apparent Volume\nof Syringe"() -> (w6588:dbl)
                                n6158 = local read "Volume of Syringe"() -> (w6590:dbl)
                                n6159 = call "RPickUp(SubVI).vi"("Volume to be picked up"=w6588, "Volume of Syringe"=w6590, "Resolution of PickUP"=w6589, "PickUp Flow Rate (ul/min)"=150.0, "VISA Refnum in"=w6591) -> ()  [unwired: 6 in, 1 out]
                                }
                                frame #1 {
                                n6160 = local read "Stopper that ends \nthe main loops"() -> (w6592:bool)
                                n6161 = local read "VISA Refnum in\nfor Pump"() -> (w6593:refnum<visa-resource-name>)
                                n6162 = case shown="True" w6592 {
                                frame False {
                                }
                                frame True {
                                n6163 = local read "VISA Refnum in\nfor Pump"() -> (w6594:refnum<visa-resource-name>)
                                n6164 = call "HardStopCurrentProcess (SubVI).vi"("VISA Refnum in"=w6594) -> ()  [unwired: 11 in]
                                }
                                }
                                n6165 = call "ProcessCompletionWaiter (SubVI).vi"("VISA Refnum in"=w6593) -> ()  [unwired: 11 in]
                                }
                                frame #2 {
                                n6166 = local read "VISA Refnum in\nfor Pump"() -> (w6596:refnum<visa-resource-name>)
                                n6167 = call "PortChanger (SubVI).vi"("Port Number"="1", "VISA Refnum in"=w6596) -> ()  [unwired: 10 in]
                                }
                                frame #3 {
                                n6168 = local read "Stopper that ends \nthe main loops"() -> (w6597:bool)
                                n6169 = local read "VISA Refnum in\nfor Pump"() -> (w6598:refnum<visa-resource-name>)
                                n6170 = case shown="True" w6597 {
                                frame False {
                                }
                                frame True {
                                n6171 = local read "VISA Refnum in\nfor Pump"() -> (w6599:refnum<visa-resource-name>)
                                n6172 = call "HardStopCurrentProcess (SubVI).vi"("VISA Refnum in"=w6599) -> ()  [unwired: 11 in]
                                }
                                }
                                n6173 = call "ProcessCompletionWaiter (SubVI).vi"("VISA Refnum in"=w6598) -> ()  [unwired: 11 in]
                                }
                                frame #4 {
                                n6174 = local read "VISA Refnum in\nfor Pump"() -> (w6604:refnum<visa-resource-name>)
                                n6175 = local read "Volume of Syringe"() -> (w6601:dbl)
                                n6176 = call "GoToAbsolutePosition(SubVI).vi"("Absolute Volume Position in Syringe (in ul)"=0.0, "Volume of Syringe"=w6601, "Resolution of Pumping"=T2."Standard Pumping", "Flow Rate (ul/min)"=150.0, "VISA Refnum in"=w6604) -> ()  [unwired: 6 in, 1 out]
                                }
                                frame #5 {
                                n6177 = local read "Stopper that ends \nthe main loops"() -> (w6605:bool)
                                n6178 = local read "VISA Refnum in\nfor Pump"() -> (w6606:refnum<visa-resource-name>)
                                n6179 = case shown="True" w6605 {
                                frame False {
                                }
                                frame True {
                                n6180 = local read "VISA Refnum in\nfor Pump"() -> (w6607:refnum<visa-resource-name>)
                                n6181 = call "HardStopCurrentProcess (SubVI).vi"("VISA Refnum in"=w6607) -> ()  [unwired: 11 in]
                                }
                                }
                                n6182 = call "ProcessCompletionWaiter (SubVI).vi"("VISA Refnum in"=w6606) -> ()  [unwired: 11 in]
                                }
                                }
                                }
                                }
                                }
                                }
                                frame #5 {
                                n6183 = local read "VISA Refnum in\nfor Pump"() -> (w6609:refnum<visa-resource-name>)
                                n6184 = local read "Port for \nB-Elution"() -> (w6608:string)
                                n6185 = call "PortChanger (SubVI).vi"("Port Number"=w6608, "VISA Refnum in"=w6609) -> ()  [unwired: 10 in]
                                }
                                frame #6 {
                                n6186 = local read "VISA Refnum in\nfor Pump"() -> (w6610:refnum<visa-resource-name>)
                                n6187 = call "ProcessCompletionWaiter (SubVI).vi"("VISA Refnum in"=w6610) -> ()  [unwired: 11 in]
                                }
                                frame #7 {
                                n6188 = local read "Buffer-B PickUp \nFlow Rate (ul/min)"() -> (w6613:dbl)
                                n6189 = local read "Buffer-B Pumping\nResolution"() -> (w6612:T2)
                                n6190 = local read "VISA Refnum in\nfor Pump"() -> (w6615:refnum<visa-resource-name>)
                                n6191 = local read "Buffer-B Volume \nto be  Pumped"() -> (w6611:dbl)
                                n6192 = local read "Volume of Syringe"() -> (w6614:dbl)
                                n6193 = call "RPickUp(SubVI).vi"("Volume to be picked up"=w6611, "Volume of Syringe"=w6614, "Resolution of PickUP"=w6612, "PickUp Flow Rate (ul/min)"=w6613, "VISA Refnum in"=w6615) -> ()  [unwired: 6 in, 1 out]
                                }
                                frame #8 {
                                n6194 = local read "Stopper that ends \nthe main loops"() -> (w6616:bool)
                                n6195 = local read "VISA Refnum in\nfor Pump"() -> (w6617:refnum<visa-resource-name>)
                                n6196 = case shown="True" w6616 {
                                frame False {
                                }
                                frame True {
                                n6197 = local read "VISA Refnum in\nfor Pump"() -> (w6618:refnum<visa-resource-name>)
                                n6198 = call "HardStopCurrentProcess (SubVI).vi"("VISA Refnum in"=w6618) -> ()  [unwired: 11 in]
                                }
                                }
                                n6199 = call "ProcessCompletionWaiter (SubVI).vi"("VISA Refnum in"=w6617) -> ()  [unwired: 11 in]
                                }
                                frame #9 {
                                # "Reads the initial Plunger Position for computing the volume dispensed"
                                n6200 = local read "VISA Refnum in\nfor Pump"() -> (w6620:refnum<visa-resource-name>)
                                n6201 = call "AbsolutePlungerPosition (SubVI).vi"("VISA Refnum in"=w6620) -> ("Plunger Position"=w6619:i32)  [unwired: 10 in]
                                n6202 = local write "Initial Plunger Position"(w6619) -> ()
                                }
                                frame #10 {
                                # "Switch to Port-2"
                                # "Port-2 of the pump is conncted to column-1 of chip"
                                n6203 = local read "VISA Refnum in\nfor Pump"() -> (w6622:refnum<visa-resource-name>)
                                n6204 = call "PortChanger (SubVI).vi"("Port Number"="2", "VISA Refnum in"=w6622) -> ()  [unwired: 10 in]
                                }
                                frame #11 {
                                n6205 = local read "Stopper that ends \nthe main loops"() -> (w6623:bool)
                                n6206 = local read "VISA Refnum in\nfor Pump"() -> (w6624:refnum<visa-resource-name>)
                                n6207 = call "ProcessCompletionWaiter (SubVI).vi"("VISA Refnum in"=w6624) -> ()  [unwired: 11 in]
                                n6208 = case shown="True" w6623 {
                                frame False {
                                }
                                frame True {
                                n6209 = local read "VISA Refnum in\nfor Pump"() -> (w6625:refnum<visa-resource-name>)
                                n6210 = call "HardStopCurrentProcess (SubVI).vi"("VISA Refnum in"=w6625) -> ()  [unwired: 11 in]
                                }
                                }
                                }
                                frame #12 {
                                # "Keeps the AMF valve after column-1 open and valve after column-2 closed"
                                n6211 = local read "VISA Refnum in\nfor Valve"() -> (w6630:refnum<visa-resource-name>)
                                n6212 = local read "External Valve \nOPEN"() -> (w6629:string)
                                n6213 = call "PortChanger_Valve (SubVI).vi"("Port Number"=w6629, "VISA Refnum in"=w6630) -> ()  [unwired: 10 in]
                                n6214 = local write "Valve V1 Open"(TRUE ("Valve V1 Open")) -> ()
                                n6215 = local write "Valve V2 Open"(TRUE ("Valve V2 Open")) -> ()
                                n6216 = local write "Valve V3 Open"(FALSE ("Valve V3 Open")) -> ()
                                n6217 = local write "Valve V4 Open"(FALSE ("Valve V4 Open")) -> ()
                                n6218 = local write "Valve V6 Open"(FALSE ("Valve V6 Open")) -> ()
                                n6219 = local write "Valve V5 Open"(FALSE ("Valve V5 Open")) -> ()
                                n6220 = local write "Valve V7 Open"(FALSE ("Valve V7 Open")) -> ()
                                }
                                frame #13 {
                                n6221 = local read "Buffer-B Dispense\nFlow Rate (ul/min)"() -> (w6640:dbl)
                                n6222 = local read "Buffer-B Pumping\nResolution"() -> (w6639:T2)
                                n6223 = local read "Initial Plunger Position"() -> (w6636:dbl)
                                n6224 = local read "VISA Refnum in\nfor Pump"() -> (w6642:refnum<visa-resource-name>)
                                n6225 = local read "Volume of Syringe"() -> (w6641:dbl)
                                n6226 = call "GoToAbsolutePosition(SubVI).vi"("Absolute Volume Position in Syringe (in ul)"=0.0 ("Volume to be Dispensed"), "Volume of Syringe"=w6641, "Resolution of Pumping"=w6639, "Flow Rate (ul/min)"=w6640, "VISA Refnum in"=w6642) -> ()  [unwired: 6 in, 1 out]
                                n6227 = local write "Pause Data Collection"(FALSE ("Pause Data Collection")) -> ()
                                n6228 = local write "Vol_now"(0.0 ("Vol_now")) -> ()
                                n6229 = local write "Position\nNow"(w6636) -> ()
                                }
                                frame #14 {
                                n6230 = while {
                                stop <- w6649 stop-if-true
                                n6231 = event shown="[0] \"Pause Elution Value\": Value Change" {
                                selector: _ -> [_ _]
                                dyn-events: _ -> [_ _]
                                timeout: 100 -> [_ _]
                                event "Pause Elution\nValue": Value Change {
                                n6232 = event-data() -> ()  [unwired: 1 in, 6 out]
                                n6233 = stacked-sequence {
                                frame #0 {
                                n6234 = local read "Pause Elution"() -> (w6651:bool)
                                n6235 = case shown="False" w6651 {
                                frame False {
                                n6236 = local write "Pause Elution"(TRUE ("Pause Elution")) -> ()
                                }
                                frame True {
                                n6237 = local write "Pause Elution"(FALSE ("Pause Elution")) -> ()
                                }
                                }
                                }
                                frame #1 {
                                n6238 = local read "Pause Elution"() -> (w6654:bool)
                                n6239 = case shown="False" w6654 {
                                frame False {
                                n6240 = local read "Buffer-B Dispense\nFlow Rate (ul/min)"() -> (w6659:dbl)
                                n6241 = local read "VISA Refnum in\nfor Pump"() -> (w6660:refnum<visa-resource-name>)
                                n6242 = local read "Buffer-B Pumping\nResolution"() -> (w6656:T2)
                                n6243 = local read "Volume of Syringe"() -> (w6657:dbl)
                                n6244 = call "GoToAbsolutePosition(SubVI).vi"("Absolute Volume Position in Syringe (in ul)"=0.0, "Volume of Syringe"=w6657, "Resolution of Pumping"=w6656, "Flow Rate (ul/min)"=w6659, "VISA Refnum in"=w6660) -> ()  [unwired: 6 in, 1 out]
                                n6245 = local write "Pause Data Collection"(FALSE ("Pause Data Collection")) -> ()
                                }
                                frame True {
                                n6246 = local read "VISA Refnum in\nfor Pump"() -> (w6662:refnum<visa-resource-name>)
                                n6247 = local write "Pause Data Collection"(TRUE ("Pause Data Collection")) -> ()
                                n6248 = call "HardStopCurrentProcess (SubVI).vi"("VISA Refnum in"=w6662) -> ()  [unwired: 11 in]
                                }
                                }
                                }
                                }
                                }
                                event Timeout {
                                n6249 = event-data() -> ()  [unwired: 1 in, 3 out]
                                }
                                }
                                n6250 = local read "Divert Sample \ninto Column-2"() -> (w6647:bool)
                                n6251 = local read "Stopper that ends \nthe main loops"() -> (w6648:bool)
                                n6252 = Or(x=w6647, y=w6648) -> (x .or. y?=w6649:bool)
                                }
                                n6253 = local read "Buffer-B Pumping\nResolution"() -> (w6645:T2)
                                n6254 = local read "VISA Refnum in\nfor Pump"() -> (w6646:refnum<visa-resource-name>)
                                n6255 = local read "Volume of Syringe"() -> (w6644:dbl)
                                n6256 = while {
                                tunnel: w6646 -> [w6671]
                                tunnel: w6645 -> [w6670]
                                tunnel: w6644 -> [w6669]
                                stop <- w6665 stop-if-true
                                n6257 = local read "Position\nNow"() -> (w6663:dbl)
